vi "Test - Shutdown Controller.vi"(8 "error in":errorcluster, 10 "Boiler Configuration":T3={"Pilot Increment (ms)"=100, "Pilot Decrement (ms)"=50}, 11 "Flame Threshold":u32=30) -> (0 "error out":errorcluster, 3 "MHL Data":T1={"Status"="Lockout", "Fuel Control Valve"=0, "Primary Fan"=FALSE, "Pilot Gas Valve"=FALSE, "Pilot"=FALSE, "Forced Draft Fan"=FALSE, "MHL Status"=enum."Lockout"})   [LabVIEW 2014, in "Controller.lvlib"]
uses:
  Controller.lvlib
  Boiler/Boiler Configuration.ctl
  controls/MHL UI Data.ctl
  controls/MHL Status.ctl
  Boiler/Boiler.lvlib
  support/Message Queue/Message Queue.lvlib
panel:
  in  "Purge Time":u32=2
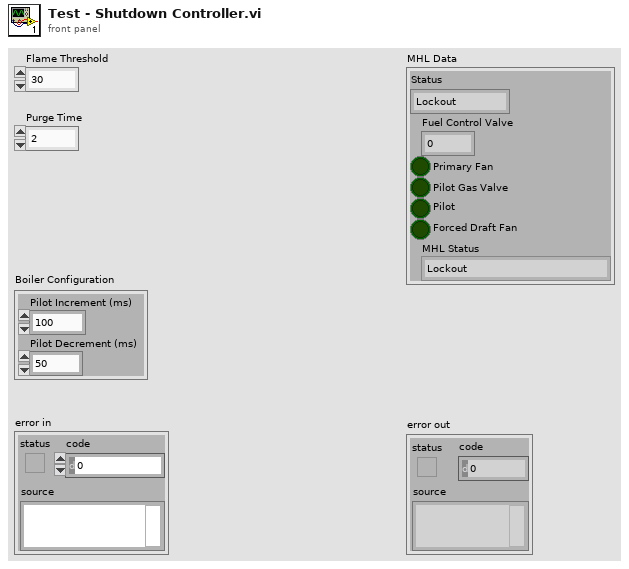
[diagram p1: front panel]
types:
  T1 = typedef "MHL UI Data.ctl" = cluster{"Status":string, "Fuel Control Valve":u32, "Primary Fan":bool, "Pilot Gas Valve":bool, "Pilot":bool, "Forced Draft Fan":bool, "MHL Status":T2}
  T2 = typedef "MHL Status.ctl" = enum16{"Lockout", "Ready", "Pre-Purge", "Pre-Purge Complete", "Pilot On", "Boiler Running", "Shutdown", "Purge"}
  T3 = typedef "Boiler.lvlib/Boiler Configuration.ctl" = cluster{"Pilot Increment (ms)":u32, "Pilot Decrement (ms)":u32}
  T4 = enum16{"open", "replace", "create", "open or create", "replace or create", "replace or create with confirmation"}
  T5 = typedef "Message Queue.lvlib/All Message Queues.ctl" = cluster{"MHL":refnum<queue>, "Boiler Controller":refnum<queue>, "Boiler":refnum<queue>}
  T6 = typedef "Notifiers.ctl" = cluster{"Handshake":refnum<notifier>, "Flame Level":refnum<notifier>, "Controller Exit":refnum<notifier>, "Boiler Exit":refnum<notifier>}
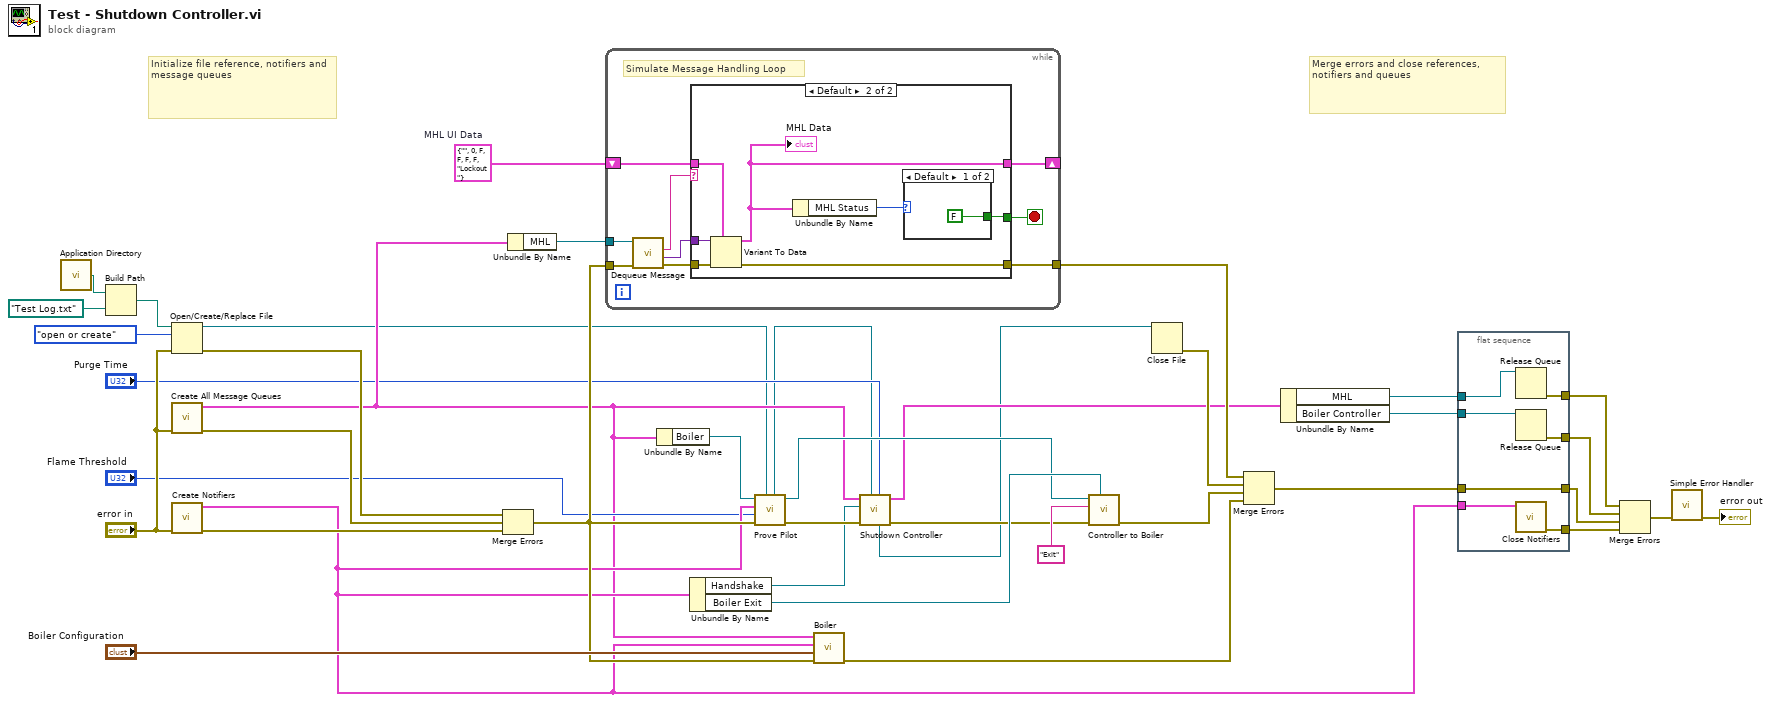
[diagram p0: block diagram]
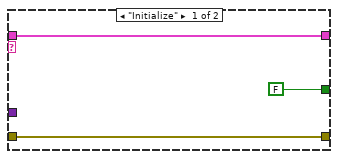
[diagram p2: hidden frame]
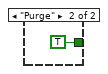
[diagram p3: hidden frame]
diagram:
  w30 = T1 {"Status"="", "Fuel Control Valve"=0, "Primary Fan"=FALSE, "Pilot Gas Valve"=FALSE, "Pilot"=FALSE, "Forced Draft Fan"=FALSE, "MHL Status"=enum."Lockout"}  # MHL UI Data
  # "Merge errors and close references, notifiers and queues"
  # "Initialize file reference, notifiers and message queues"
  n1 = call <vilib>:"Application Directory.vi"() -> ("Application Directory"=w38:path)
  n2 = Build Path(base path=w38, name or relative path=path "Test Log.txt") -> (appended path=w36:path)
  n3 = Open/Create/Replace File(file path (use dialog)=w36, error in="error in", operation (0:open)=T4."open or create") -> (refnum out=w2:refnum<file>, error out=w34:errorcluster)  [unwired: 3 in, 1 out]
  n4 = call "Create All Message Queues.vi"("error in"="error in") -> ("error out"=w39:errorcluster, "Message Queues out"=w7:T5)  [unwired: 9 in]
  n5 = call "Create Notifiers.vi"("error in"="error in") -> ("error out"=w40:errorcluster, "Notifiers"=w13:T6)  [unwired: 9 in]
  n6 = Merge Errors(w34, w39, w40) -> (w14:errorcluster)
  n7 = Unbundle By Name(w7) -> ("MHL"=w31:refnum<queue>)
  n8 = while {
    tunnel: w31 -> [w49]
    tunnel: w14 -> [w48]
    shift-right: [w45] -> _
    shift-left: w30 -> [w46]
    tunnel: [w42] -> w26
    stop <- w41 stop-if-true
    # "Simulate Message Handling Loop"
    n9 = call "Dequeue Message.vi"("error in (no error)"=w48, "Message Queue"=w49) -> ("error out"=w43:errorcluster, "Message Data"=w47:variant, "Message"=w44:string)  [unwired: 6 in, 1 out]
    n10 = case shown="Default" w44 {
      tunnel: w43 -> [w50 w59]
      tunnel: w47 -> [_ w58]
      tunnel: w46 -> [w52 w57]
      tunnel: [w52 w56] -> w45
      tunnel: [FALSE w54] -> w41
      tunnel: [w50 w53] -> w42
      frame "Initialize" {
      }
      frame Default {
        n11 = Variant To Data(error in=w59, type=w57, Variant=w58) -> (data=w56:T1, error out=w53:errorcluster)
        "MHL Data" <- w56
        n12 = Unbundle By Name(w56) -> ("MHL Status"=w55:T2)
        n13 = case shown="Default" w55 {
          tunnel: [FALSE TRUE] -> w54
          frame Default {
          }
          frame "Purge" {
          }
        }
      }
    }
  }
  n14 = Unbundle By Name(w7) -> ("Boiler"=w11:refnum<queue>)
  n15 = Unbundle By Name(w13) -> ("Handshake"=w5:refnum<notifier>, "Boiler Exit"=w20:refnum<notifier>)
  n16 = call "Prove Pilot.vi"("Log File Refnum in"=w2, "error in"=w14, "Flame Threshold"="Flame Threshold", "Notifiers in"=w13, "Boiler Queue in"=w11) -> ("error out"=w9:errorcluster, "Boiler Queue out"=w10:refnum<queue>, "Log File Refnum out"=w1:refnum<file>)  [unwired: 3 in, 1 out]
  n17 = call "Boiler.vi"("error in"=w14, "Boiler Configuration"="Boiler Configuration", "Notifiers"=w13, "Message Queues"=w7) -> ("error out"=w16:errorcluster)  [unwired: 7 in]
  n18 = call "Shutdown Controller.vi"("Purge Time"="Purge Time", "Log File Refnum in"=w1, "error in"=w9, "Handshake Notifier in"=w5, "Message Queues in"=w7) -> ("error out"=w8:errorcluster, "Message Queues out"=w6:T5, "Log File Refnum out"=w3:refnum<file>)  [unwired: 2 in, 2 out]
  n19 = call "Controller to Boiler.vi"("Notifier"=w20, "error in"=w8, "Message"="Exit", "Boiler Queue in"=w10) -> ("error out"=w15:errorcluster)  [unwired: 5 in, 2 out]
  n20 = Close File(refnum=w3) -> (error out=w27:errorcluster)  [unwired: 1 in, 1 out]
  n21 = Merge Errors(w26, w27, w15, w16) -> (w17:errorcluster)
  n22 = Unbundle By Name(w6) -> ("MHL"=w28:refnum<queue>, "Boiler Controller"=w29:refnum<queue>)
  n23 = flat-sequence {
    tunnel: w29 -> [w68]
    tunnel: w28 -> [w67]
    tunnel: [w66] -> w24
    tunnel: [w65] -> w23
    tunnel: [w64] -> w19
    tunnel: w13 -> [w63]
    tunnel: [w62] -> w18
    tunnel: w17 -> [w62]
    frame #0 {
      n24 = Release Queue(queue=w67) -> (error out=w65:errorcluster)  [unwired: 2 in, 2 out]
      n25 = Release Queue(queue=w68) -> (error out=w66:errorcluster)  [unwired: 2 in, 2 out]
      n26 = call "Close Notifiers.vi"("Notifiers"=w63) -> ("error out"=w64:errorcluster)  [unwired: 10 in]
    }
  }
  n27 = Merge Errors(w23, w24, w18, w19) -> (w22:errorcluster)
  n28 = call <vilib>:"Simple Error Handler.vi"("error in (no error)"=w22) -> ("error out"=→"error out":errorcluster)  [unwired: 4 in, 4 out]
